vi "SubVI_Classificador_de_forma_3.vi"(8 "error in":errorcluster, 10 "ROI Objeto":T3 {"Contours"."Type" items=["No Selection", "Point", "Line", "Rectangle", "Oval", "Polygon", "Free", "Annulus", "Unused2", "Unused3", "Broken Line", "Free Hand Line", "Rotated Rectangle"]}, 11 "Session In":T2) -> (0 "error out":errorcluster, 1 "Points":cluster{"X":dbl, "Y":dbl}[](array[cluster]), 2 "Forma":string, 3 "Session Out":T2)   [LabVIEW 2017]
uses:
  <vilib>/userdefined/High Color/IMAQdx.ctl
  <vilib>/vision/driver/IMAQdx.llb/IMAQdx Buffer Number Mode.ctl
  <vilib>/vision/driver/NI_Vision_Acquisition_Software.lvlib
  <vilib>/vision/NI_Vision_Development_Module.lvlib
panel:
  out "Imagem 4":T1(plugin-control)
  out "Imagem2":T1(plugin-control)
  out "Imagem 3":T1(plugin-control)
  out "Imagem1":T1(plugin-control)
  out "Imagem Original":T1(plugin-control)
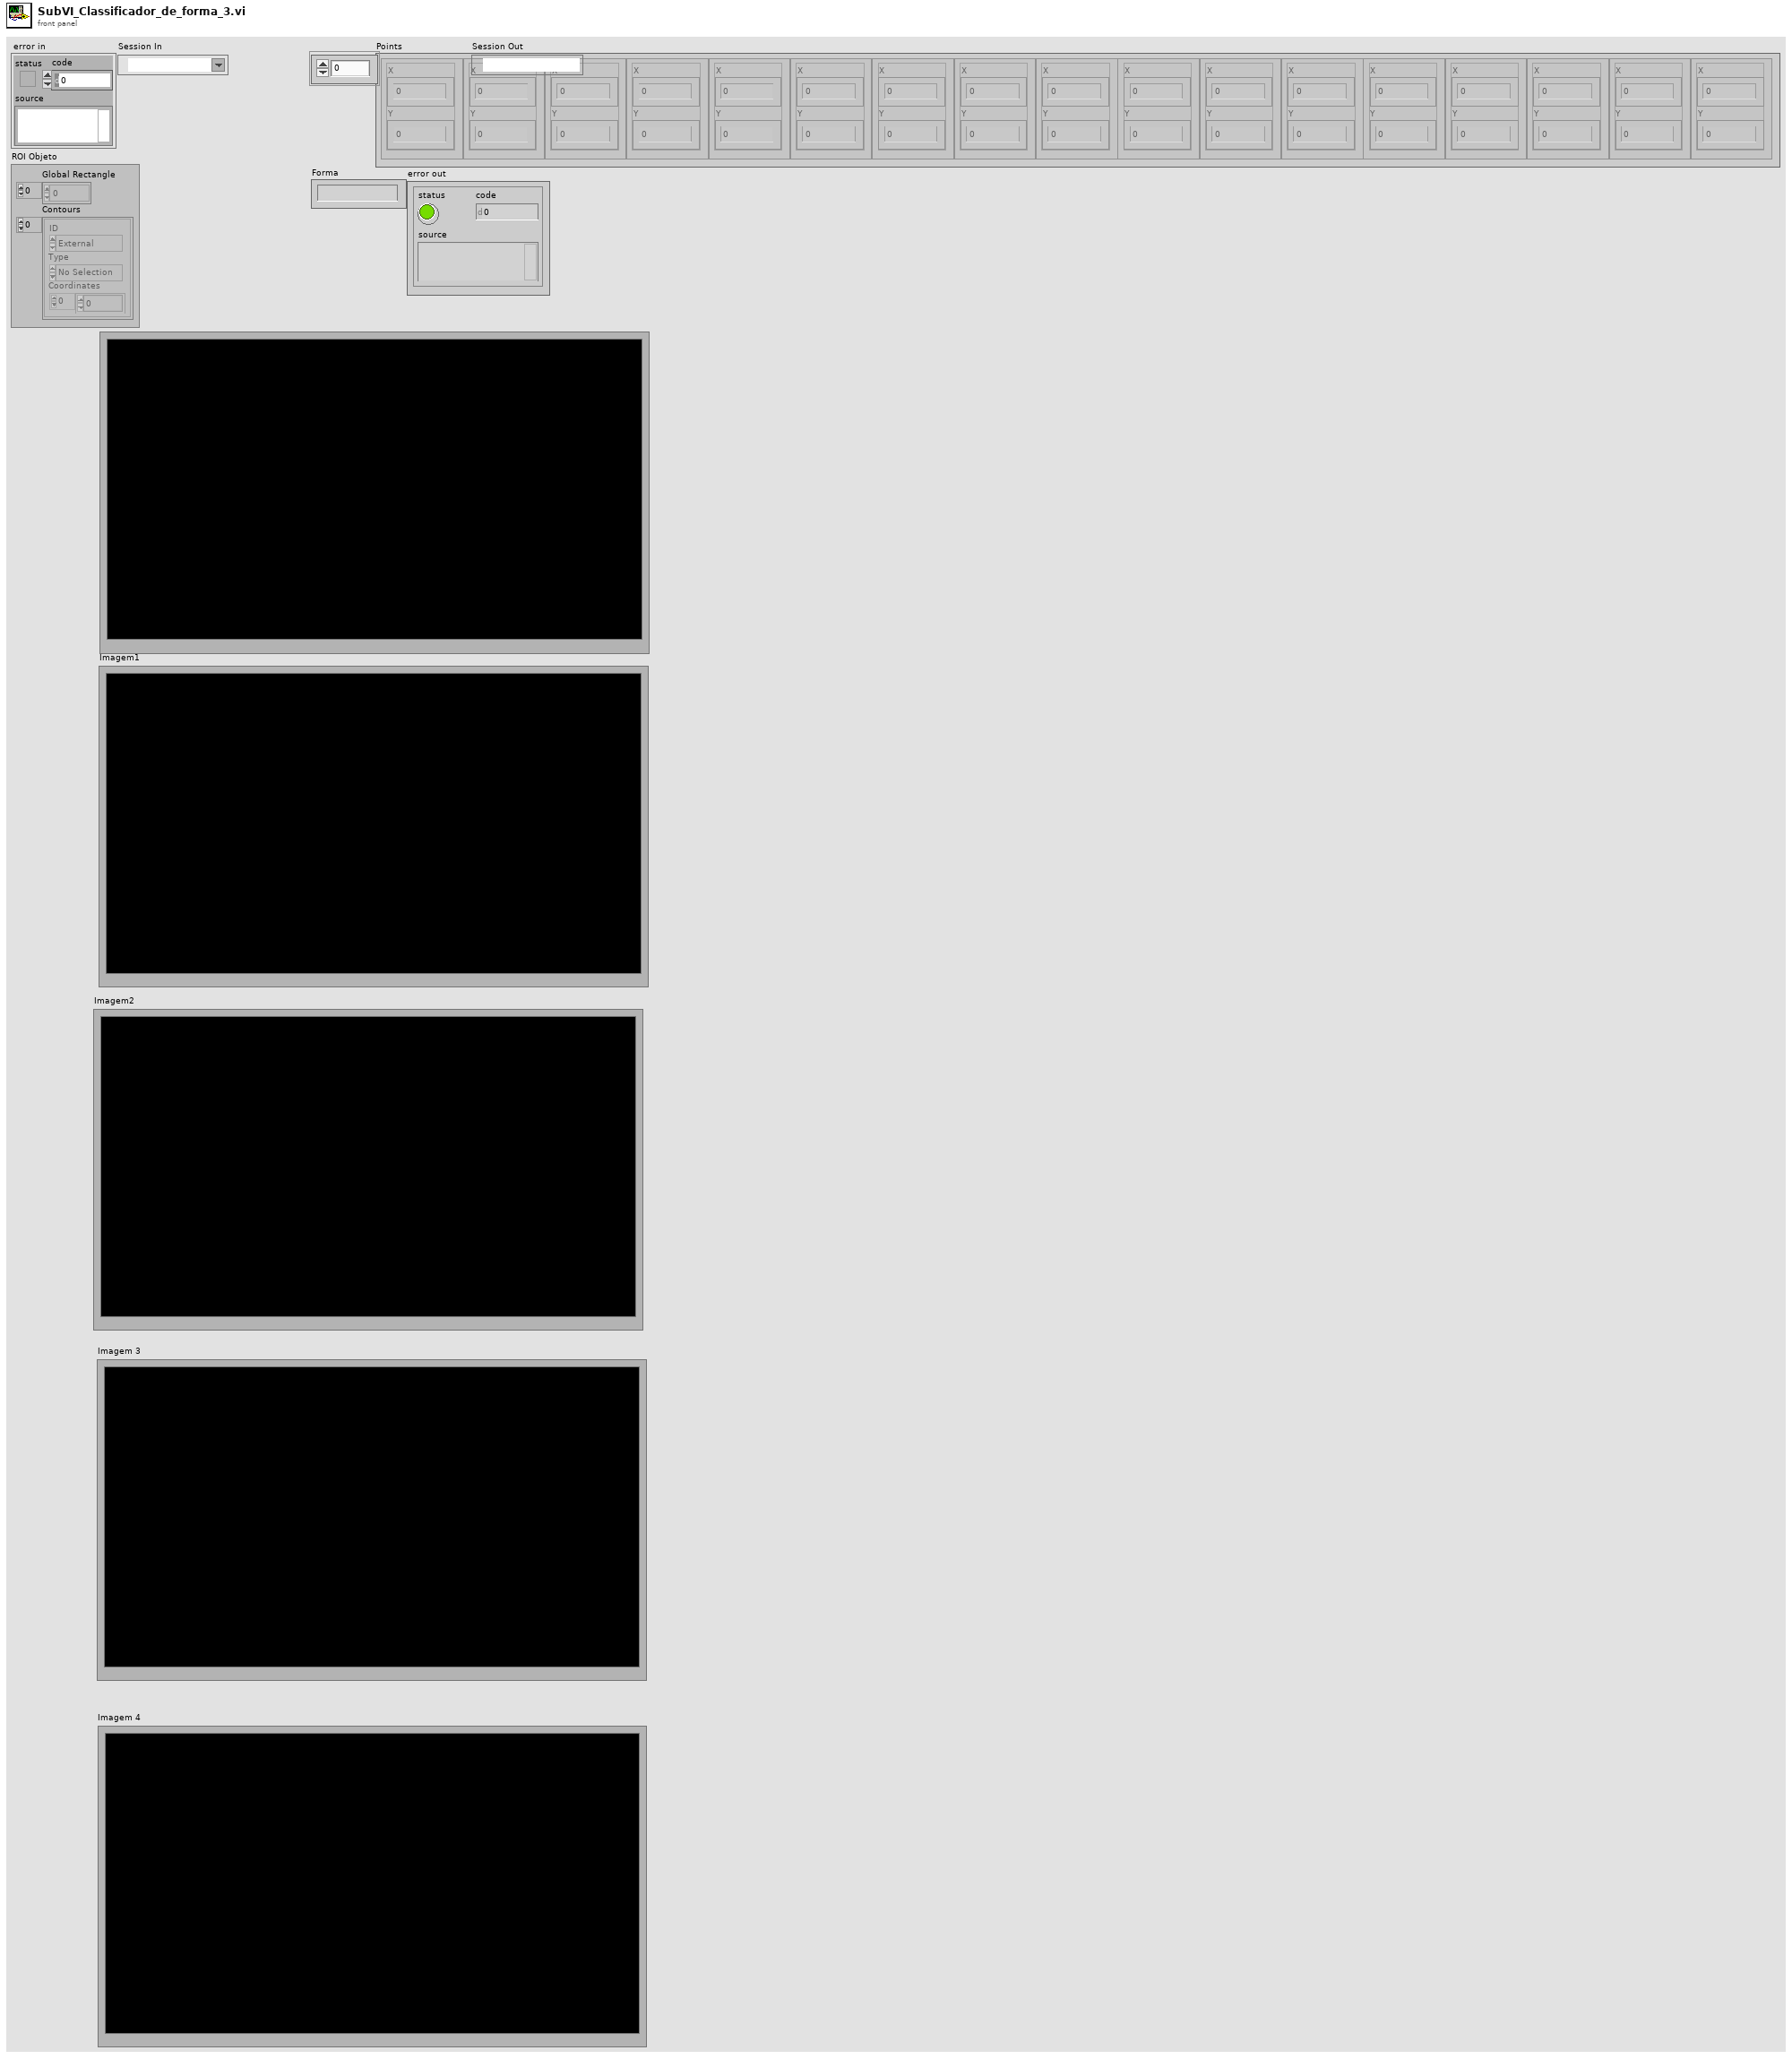
[diagram p1: front panel]
types:
  T1 = typedef "IMAQ Image.ctl" = refnum<image>
  T2 = typedef "IMAQdx.ctl" = refnum<k21>
  T3 = cluster{"Global Rectangle":i32[], "Contours":cluster{"ID":enum32{"External", "Internal"}, "Type":u32, "Coordinates":i32[]}[]}
  T4 = typedef "Image Type" = u32
  T5 = enum32{"AutoM", "Close", "Dilate", "Erode", "Gradient", "Gradient out", "Gradient in", "Hit miss", "Open", "PClose", "POpen", "Thick", "Thin"}
  T6 = typedef "NI_Vision_Acquisition_Software.lvlib/IMAQdx Buffer Number Mode.ctl" = enum32{"Next", "Last", "Buffer Number", "Every", "Last New"}
  T7 = typedef "IMAQ ExtractCurvesCurve.ctl" = cluster{"Points":cluster{"X":dbl, "Y":dbl}[], "Closed?":bool, "Curve Length":dbl, "Min Edge Strength":dbl, "Max Edge Strength":dbl, "Average Edge Strength":dbl}
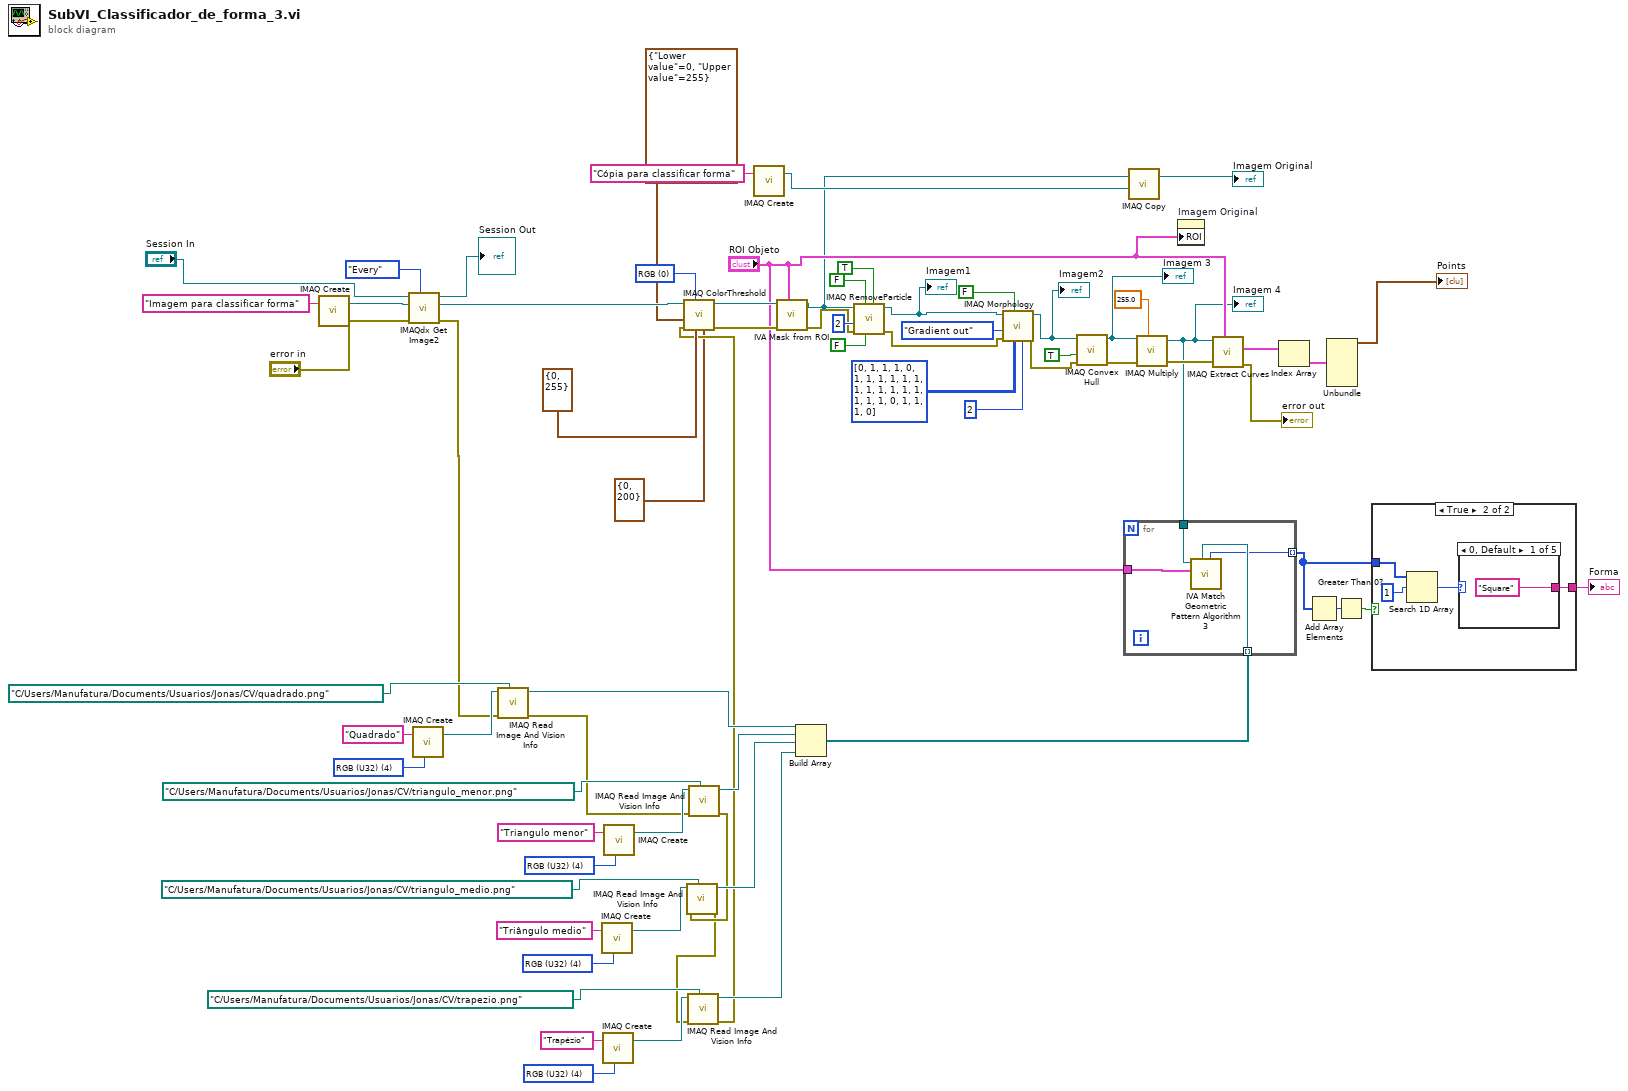
[diagram p0: block diagram]
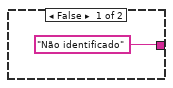
[diagram p2: hidden frame]
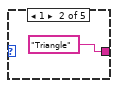
[diagram p3: hidden frame]
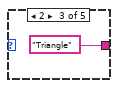
[diagram p4: hidden frame]
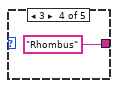
[diagram p5: hidden frame]
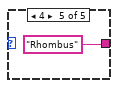
[diagram p6: hidden frame]
diagram:
  w35 = T4 4 items=["Grayscale (U8)", "Grayscale (I16)", "Grayscale (SGL)", "Complex (CSG)", "RGB (U32)", "HSL (U32)", "RGB (U64)", "Grayscale (U16)"] ("Image Type")
  w40 = T4 4 items=["Grayscale (U8)", "Grayscale (I16)", "Grayscale (SGL)", "Complex (CSG)", "RGB (U32)", "HSL (U32)", "RGB (U64)", "Grayscale (U16)"] ("Image Type")
  w43 = T4 4 items=["Grayscale (U8)", "Grayscale (I16)", "Grayscale (SGL)", "Complex (CSG)", "RGB (U32)", "HSL (U32)", "RGB (U64)", "Grayscale (U16)"] ("Image Type")
  w48 = T4 4 items=["Grayscale (U8)", "Grayscale (I16)", "Grayscale (SGL)", "Complex (CSG)", "RGB (U32)", "HSL (U32)", "RGB (U64)", "Grayscale (U16)"] ("Image Type")
  w66 = u16 0 items=["RGB", "HSL", "HSV", "HSI"] ("Color Mode")
  n1 = call "IMAQ Create"("Image Name"="Imagem para classificar forma") -> ("New Image"=w69:T1)  [unwired: 4 in, 1 out]
  n2 = call <vilib>:"IMAQdx Get Image2.vi"("Buffer Number Mode (Next)"=IMAQdx_Buffer_Number_Mode."Every", "error in"="error in", "Image In"=w69, "Session In"="Session In") -> ("error out"=w17:errorcluster, "Image Out"=w67:T1, "Session Out"=→"Session Out":T2)  [unwired: 4 in, 1 out]
  n3 = call "IMAQ Create"("Image Name"="Quadrado", "Image Type"=w48) -> ("New Image"=w47:T1)  [unwired: 3 in, 1 out]
  n4 = call "IMAQ Read Image And Vision Info"("File Path"=path "C:/Users/Manufatura/Documents/Usuarios/Jonas/CV/quadrado.png" ("Template File Path"), "error in (no error)"=w17, "Image"=w47) -> ("error out"=w16:errorcluster, "Image Out"=w33:T1)  [unwired: 1 in, 6 out]
  n5 = call "IMAQ Create"("Image Name"="Triângulo medio", "Image Type"=w43) -> ("New Image"=w44:T1)  [unwired: 3 in, 1 out]
  n6 = call "IMAQ Create"("Image Name"="Trapézio", "Image Type"=w40) -> ("New Image"=w39:T1)  [unwired: 3 in, 1 out]
  n7 = call "IMAQ Create"("Image Name"="Triangulo menor", "Image Type"=w35) -> ("New Image"=w36:T1)  [unwired: 3 in, 1 out]
  n8 = call "IMAQ Read Image And Vision Info"("File Path"=path "C:/Users/Manufatura/Documents/Usuarios/Jonas/CV/triangulo_menor.png" ("Template File Path"), "error in (no error)"=w16, "Image"=w36) -> ("error out"=w15:errorcluster, "Image Out"=w32:T1)  [unwired: 1 in, 6 out]
  n9 = call "IMAQ Read Image And Vision Info"("File Path"=path "C:/Users/Manufatura/Documents/Usuarios/Jonas/CV/triangulo_medio.png" ("Template File Path"), "error in (no error)"=w15, "Image"=w44) -> ("error out"=w14:errorcluster, "Image Out"=w31:T1)  [unwired: 1 in, 6 out]
  n10 = call "IMAQ Read Image And Vision Info"("File Path"=path "C:/Users/Manufatura/Documents/Usuarios/Jonas/CV/trapezio.png" ("Template File Path"), "error in (no error)"=w14, "Image"=w39) -> ("error out"=w13:errorcluster, "Image Out"=w30:T1)  [unwired: 1 in, 6 out]
  n11 = call "IMAQ ColorThreshold"("Blue or Luma or Val or Inten Range"=cluster{"Lower value":i32, "Upper value":i32} {"Lower value"=0, "Upper value"=200}, "Green or Sat Range"=cluster{"Lower value":i32, "Upper value":i32} {"Lower value"=0, "Upper value"=255}, "Color Mode"=w66, "error in (no error)"=w13, "Red or Hue Range"=cluster{"Lower value":i32, "Upper value":i32} {"Lower value"=0, "Upper value"=255}, "Image Src"=w67) -> ("error out"=w26:errorcluster, "Image Dst Out"=w63:T1)  [unwired: 2 in, 2 out]
  n12 = call "IMAQ Create"("Image Name"="Cópia para classificar forma") -> ("New Image"=w7:T1)  [unwired: 4 in, 1 out]
  n13 = call <vilib>:"IVA Mask from ROI.vi"("ROI Descriptor"="ROI Objeto", "error in (no error)"=w26, "Image Src"=w63) -> ("error out"=w25:errorcluster, "Image Out"=w6:T1)  [unwired: 2 in, 5 out]
  n14 = Build Array(w33, w32, w31, w30) -> (w29:T1[])
  n15 = call "IMAQ RemoveParticle"("Connectivity 4/8 (8)"=TRUE, "Low Pass/High Pass (Low)"=FALSE, "Square/Hexa (Square)"=FALSE, "error in (no error)"=w25, "Number of Erosion"=2, "Image Src"=w6) -> ("error out"=w24:errorcluster, "Image Dst Out"=w4:T1)  [unwired: 1 in, 3 out]
  "Imagem1" <- w4
  n16 = call "IMAQ Morphology"("Number of iterations (1)"=2, "Structuring Element"=i32[][] [[0, 1, 1, 1, 0], [1, 1, 1, 1, 1], [1, 1, 1, 1, 1], [1, 1, 1, 1, 1], [0, 1, 1, 1, 0]], "Square/Hexa (Square)"=FALSE, "error in (no error)"=w24, "Operation"=T5."Gradient out", "Image Src"=w4) -> ("error out"=w23:errorcluster, "Image Dst Out"=w3:T1)  [unwired: 1 in, 3 out]
  "Imagem2" <- w3
  n17 = call "IMAQ Convex Hull"("error in (no error)"=w23, "Connectivity 4/8 (8)"=TRUE, "Image Src"=w3) -> ("error out"=w22:errorcluster, "Image Dst Out"=w2:T1)  [unwired: 1 in, 6 out]
  "Imagem 3" <- w2
  n18 = call "IMAQ Copy"("Image Dst"=w7, "Image Src"=w6) -> ("Image Dst Out"=→"Imagem Original":T1)  [unwired: 4 in, 1 out]
  n19 = call "IMAQ Multiply"("Image Src A"=w2, "Constant"=255.0, "error in (no error)"=w22) -> ("Image Dst Out"=w1:T1, "error out"=w18:errorcluster)  [unwired: 4 in]
  "Imagem 4" <- w1
  n20 = for {
    tunnel: w29 -> [w73] mode=indexing
    tunnel: "ROI Objeto" -> [w75]
    tunnel: w1 -> [w74]
    tunnel: [w72] -> w20 mode=indexing
    n21 = call <vilib>:"IVA Match Geometric Pattern Algorithm 3.vi"("Template"=w73, "ROI Descriptor"=w75, "Image"=w74) -> ("Number of Matches"=w72:i32)  [unwired: 2 in, 6 out]
  }
  n22 = property on="Imagem Original" class="ImageControl"("ROI"="ROI Objeto") -> ()  [unwired: 2 in, 2 out]
  n23 = call "IMAQ Extract Curves"("ROI Descriptor"="ROI Objeto", "error in (no error)"=w18, "Image"=w1) -> ("error out"=→"error out":errorcluster, "Curves"=w51:T7[])  [unwired: 6 in, 1 out]
  n24 = Index Array(array=w51) -> (element=w52:T7)  [unwired: 1 in]
  n25 = Add Array Elements(numeric array=w20) -> (sum=w21:i32)
  n26 = Unbundle(w52) -> ("Points"=→"Points":cluster{"X":dbl, "Y":dbl}[])  [unwired: 5 out]
  n27 = Greater Than 0?(x=w21) -> (x > 0?=w19:bool)
  n28 = case shown="True" w19 {
    tunnel: w20 -> [_ w80]
    tunnel: ["Não identificado" w77] -> w28
    frame False {
    }
    frame True {
      n29 = Search 1D Array(1D array=w80, element=1) -> (index of element=w78:i32)  [unwired: 1 in]
      n30 = case shown="0, Default" w78 {
        tunnel: ["Square" "Triangle" "Triangle" "Rhombus" "Rhombus"] -> w77
        frame 0, Default {
        }
        frame 1 {
        }
        frame 2 {
        }
        frame 3 {
        }
        frame 4 {
        }
      }
    }
  }
  "Forma" <- w28
